vi "基于延迟的串口通信流程(组件编程）.vi"() -> ()   [LabVIEW 2013]
panel:
  out "读取缓冲区":string
  in  "查询":string(combo)="CH0"
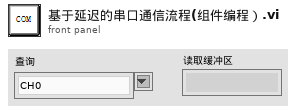
[diagram p1: front panel]
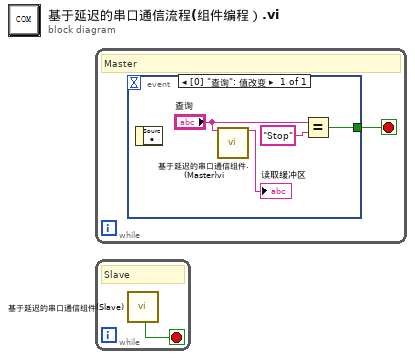
[diagram p0: block diagram]
diagram:
  n1 = while {
    stop <- w1 stop-if-true
    # "Master"
    n2 = event shown="[0] \"查询\": 值改变" {
      selector: _ -> [_]
      dyn-events: _ -> [_]
      timeout: _ -> [_]
      tunnel: [w4] -> w1
      event "查询": Value Change {
        n3 = event-data() -> ()  [unwired: 1 in, 1 out]
        n4 = call "基于延迟的串口通信组件.(Master)vi.vi"("查询"="查询") -> ("读取缓冲区"=→"读取缓冲区":string)  [unwired: 17 in, 1 out]
        n5 = Equal?(x="查询", y="Stop") -> (x = y?=w4:bool)
      }
    }
  }
  n6 = while "While循环" {
    stop <- w6 stop-if-true
    # "Slave"
    n7 = call "基于延迟的串口通信组件(Slave).vi"() -> ("Stop"=w6:bool)  [unwired: 18 in, 1 out]
  }
